vi "keithley-2450_max_p_list.vi"(0 "VISA resource name in":refnum<visa-resource-name>, 11 "Voltage List":dbl[](array[numeric])) -> (4 "VISA resource name out":refnum<visa-resource-name>, 6 "Data Array":dbl[][](array[numeric]), 15 "Measurement Complete":bool)   [LabVIEW 2016]
doc: "Configures a sweep and takes voltage and current readings at each point."
uses:
  <instrlib>/Keithley 2450/Keithley 2450.lvlib
panel:
  in  "Source Mode  (0: Voltage)":u16(ring) items=["Voltage", "Current"]
  # "(c) 2006 National Instruments.  ALL RIGHTS RESERVED."
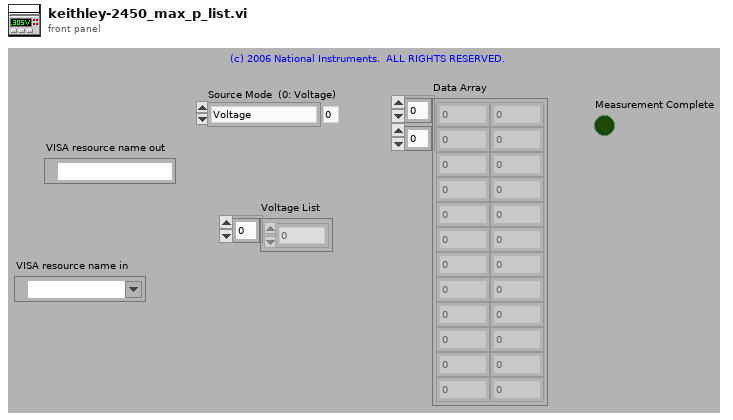
[diagram p1: front panel]
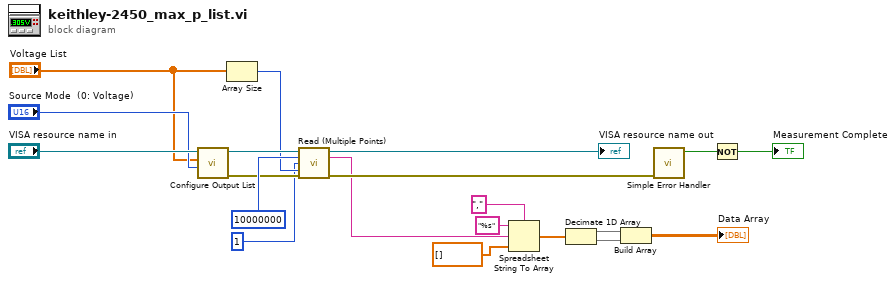
[diagram p0: block diagram]
diagram:
  n1 = call <instrlib>:"Configure Output List.vi"("Source Mode  (0: Voltage)"="Source Mode  (0: Voltage)", "Output List"="Voltage List", "VISA resource name"="VISA resource name in") -> ("error out"=w14:errorcluster, "VISA resource name out"=w15:refnum<visa-resource-name>)  [unwired: 7 in]
  n2 = Array Size(array="Voltage List") -> (size(s)=w10:i32)
  n3 = call <instrlib>:"Read (Multiple Points).vi"("VISA resource name"=w15, "Timeout (10000 ms)"=10000000, "Start Index (1)"=1, "End Index (1)"=w10, "error in (no error)"=w14) -> ("VISA resource name out"=→"VISA resource name out":refnum<visa-resource-name>, "Data out"=w2:string, "error out"=w20:errorcluster)  [unwired: 8 in]
  n4 = Spreadsheet String To Array(delimiter (Tab)=",", format string="%s", spreadsheet string=w2, array type (2D Dbl)=dbl[] []) -> (array=w5:dbl[])
  n5 = Decimate 1D Array(w5) -> (w4:dbl[], w3:dbl[])
  n6 = Build Array(w4, w3) -> (→"Data Array":dbl[][])
  n7 = call <vilib>:"Simple Error Handler.vi"("error in (no error)"=w20) -> ("error?"=w18:bool)  [unwired: 4 in, 4 out]
  n8 = Not(x=w18) -> (.not. x?=→"Measurement Complete":bool)
